vi "Set Type Code.vi"(8 "error in (no error)":errorcluster, 10 "Type":T1, 11 "LVType.lvclass in":refnum<class "LVType.lvclass">) -> (0 "error out":errorcluster, 3 "LVType.lvclass out":refnum<class "LVType.lvclass">)   [LabVIEW 2020, in "LVDataTypes.lvlib" / "LVType.lvclass"]
uses:
  <vilib>/AppBuilder/Engine/WebServiceDescription/LVDataTypes/LVType/LVType.lvclass
  <vilib>/AppBuilder/Engine/WebServiceDescription/LVDataTypes/TypeCode.ctl
  <vilib>/AppBuilder/Engine/WebServiceDescription/LVDataTypes/LVType/LVType.lvclass/LVType.ctl
  <vilib>/AppBuilder/Engine/WebServiceDescription/LVDataTypes/LVDataTypes.lvlib
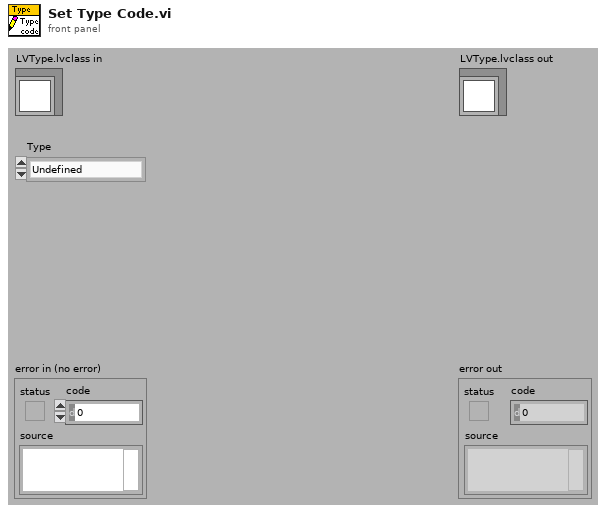
[diagram p1: front panel]
types:
  T1 = typedef "LVDataTypes.lvlib/TypeCode.ctl" = enum16{"Undefined", "Byte", "Unsigned Byte", "Word", "Unsigned Word", "Long", "Unsigned Long", "Quad", "Unsigned Quad", "Single", "Double", "Extended", "Enum", "Boolean", "String", "Path", "Array", "Cluster", "AnalogWaveform", "DigitalWaveform", "Time Stamp", "Void", "Complex Single", "Complex Double", "Complex Extended"}
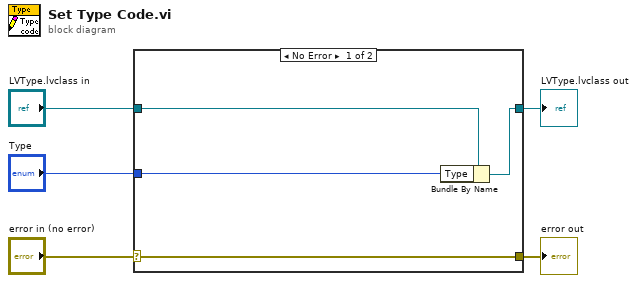
[diagram p0: block diagram]
diagram:
  n1 = case shown="No Error" "error in (no error)" {
    selector: "error in (no error)" -> [w9 w10]
    tunnel: [w9 w10] -> w4
    tunnel: [w7 w11] -> w2
    tunnel: "LVType.lvclass in" -> [w8 w11]
    tunnel: "Type" -> [w6 _]
    frame No Error {
      n2 = Bundle By Name(cluster=w8, "Type"=w6) -> (w7:refnum<class "LVType.lvclass">)
    }
    frame Error {
    }
  }
  "error out" <- w4
  "LVType.lvclass out" <- w2
